vi "Event Structure Support in LabVIEW Real-Time.vi"() -> ()   [LabVIEW 2019]
panel:
  out "Numeric Indicator within Event":i32
  in  "stop":bool
  out "event loop iteration":i32
  out "error out":errorcluster
  in  "Numeric":i32
  out "nonevent loop iteration":i32
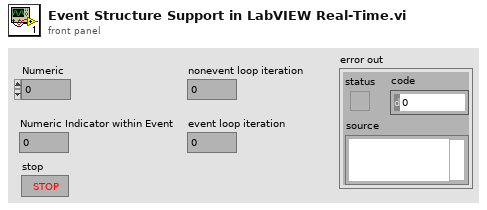
[diagram p1: front panel]
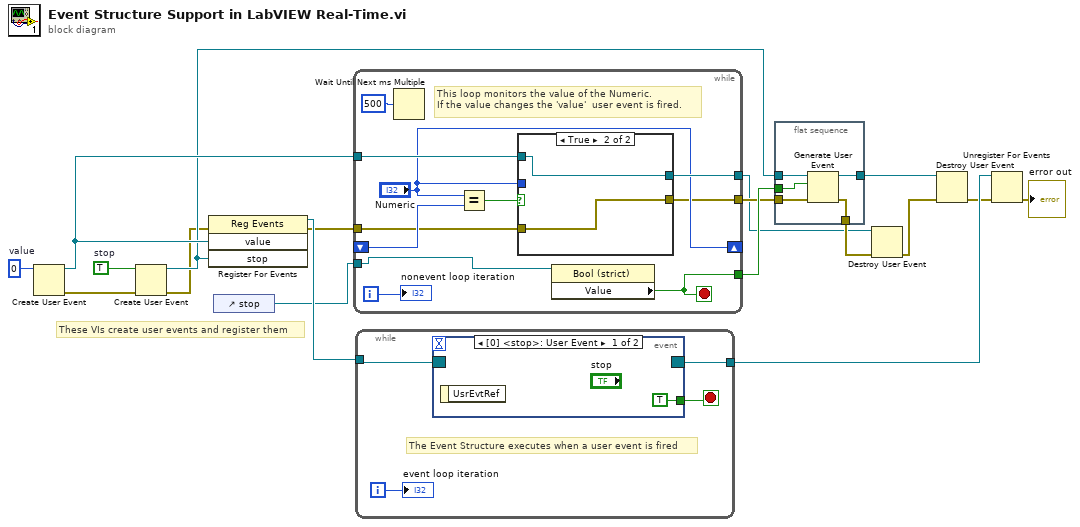
[diagram p0: block diagram]
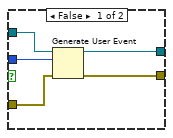
[diagram p2: hidden frame]
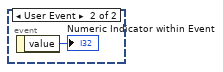
[diagram p3: hidden frame]
diagram:
  w13 = TRUE  # stop
  w16 = 0  # value
  # "These VIs create user events and register them"
  n1 = Create User Event(user event datatype=w16) -> (user event=w17:refnum<user-event>, error out=w7:errorcluster)  [unwired: 1 in]
  n2 = Create User Event(user event datatype=w13, error in=w7) -> (user event=w12:refnum<user-event>, error out=w6:errorcluster)
  n3 = register-events(error in=w6, w17, w12) -> (reference out=w18:refnum<event-registration>, error out=w5:errorcluster)  [unwired: 1 in]
  n4 = control-ref of="stop"() -> (w1:refnum<vi>)
  n5 = while {
    shift-right: ["Numeric"] -> _
    shift-left: _ -> [w26]
    tunnel: w17 -> [w25]
    tunnel: [w24] -> w2
    tunnel: [w23] -> w8
    tunnel: w5 -> [w21]
    tunnel: [w20] -> w4
    tunnel: w1 -> [w19]
    i -> [w27]
    stop <- w23 stop-if-true
    # "This loop monitors the value of the Numeric.\nIf the value changes the 'value'  user event is fired."
    n6 = Wait Until Next ms Multiple(millisecond multiple=u32 500) -> ()  [unwired: 1 out]
    n7 = Equal?(x="Numeric", y=w26) -> (x = y?=w28:bool)
    n8 = case shown="True" w28 {
      tunnel: "Numeric" -> [w33 _]
      tunnel: w25 -> [w34 w36]
      tunnel: [w32 w36] -> w24
      tunnel: w21 -> [w31 w35]
      tunnel: [w30 w35] -> w20
      frame False {
        n9 = Generate User Event(user event=w34, event data cluster=w33, error in=w31) -> (user event out=w32:refnum<user-event>, error out=w30:errorcluster)  [unwired: 1 in]
      }
      frame True {
      }
    }
    n10 = property class="Bool (strict)"(reference=w19) -> ("Value"=w23:bool)  [unwired: 1 in, 2 out]
    "nonevent loop iteration" <- w27
  }
  n11 = while {
    tunnel: w18 -> [w38]
    tunnel: [w37] -> w15
    i -> [w39]
    stop <- w40 stop-if-true
    # "The Event Structure executes when a user event is fired"
    n12 = event shown="[0] <stop>: User Event" {
      selector: w38 -> [_ _]
      dyn-events: [_ _] -> w37
      timeout: _ -> [_ _]
      tunnel: [TRUE ("stop") _] -> w40
      event User Event {
        n13 = event-data() -> ()  [unwired: 1 in, 1 out]
      }
      event User Event {
        n14 = event-data() -> ("value"=→"Numeric Indicator within Event":i32)  [unwired: 1 in]
      }
    }
    "event loop iteration" <- w39
  }
  n15 = flat-sequence {
    tunnel: w12 -> [w47]
    tunnel: [w46] -> w9
    tunnel: w8 -> [w45]
    tunnel: w4 -> [w44]
    tunnel: [w43] -> w3
    frame #0 {
      n16 = Generate User Event(user event=w47, event data cluster=w45, error in=w44) -> (user event out=w46:refnum<user-event>, error out=w43:errorcluster)  [unwired: 1 in]
    }
  }
  n17 = Destroy User Event(user event=w2, error in=w3) -> (error out=w11:errorcluster)
  n18 = Destroy User Event(user event=w9, error in=w11) -> (error out=w10:errorcluster)
  n19 = Unregister For Events(event registration refnum=w15, error in=w10) -> (error out=→"error out":errorcluster)
